vi "Set Decimation.vi"(8 "error in":errorcluster, 10 "decimation":i32, 11 "custom device ref":T1 format="%.0x") -> (0 "error out":errorcluster, 3 "custom device ref out":T1 format="%.0x")   [LabVIEW 2020, in "AIM ARINC 664 Scripting.lvlib"]
uses:
  AIM ARINC 664 Scripting.lvlib
  <vilib>/NI VeriStand/Custom Device API/Custom Device API.lvlib
  <vilib>/NI VeriStand/Custom Device API/Custom Device Item Ref.ctl
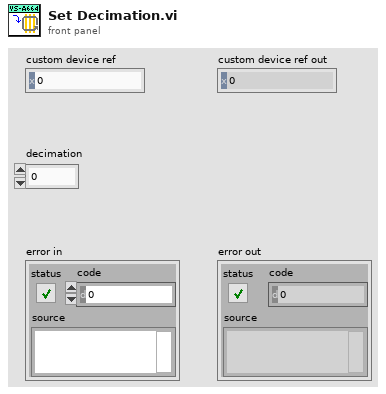
[diagram p1: front panel]
types:
  T1 = typedef "Custom Device API.lvlib/Custom Device Item Ref.ctl" = u64
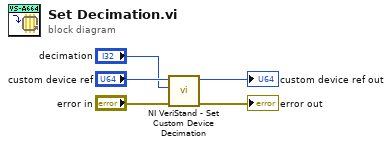
[diagram p0: block diagram]
diagram:
  n1 = call <vilib>:"NI VeriStand - Set Custom Device Decimation.vi"("error in (no error)"="error in", "Decimation"="decimation", "Device Ref in"="custom device ref") -> ("error out"=→"error out":errorcluster, "Device Ref out"=→"custom device ref out":T1)  [unwired: 7 in]
